vi "fgv_udp_remote.vi"(7 "cmd":enum16{"init", "read", "write", "close"}(ring), 8 "error in":errorcluster, 10 "send data":string) -> (0 "error out":errorcluster, 3 "receive":string)   [LabVIEW 2019]
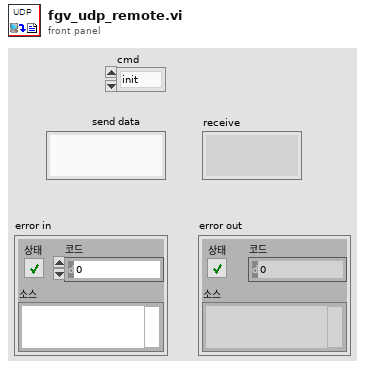
[diagram p1: front panel]
types:
  T1 = cluster{"local port":u16, "remote port":u16, "RBA IP":string}
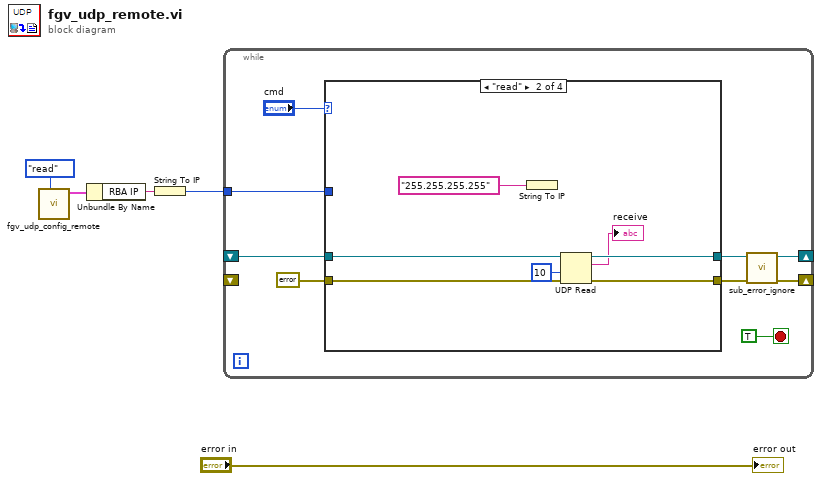
[diagram p0: block diagram]
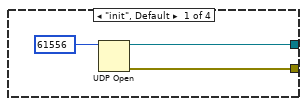
[diagram p2: hidden frame]
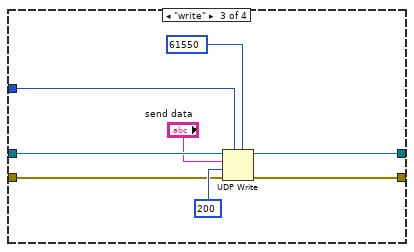
[diagram p3: hidden frame]
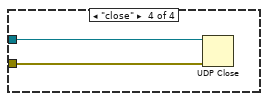
[diagram p4: hidden frame]
diagram:
  n1 = call "fgv_udp_config_remote.vi"("cmd"=enum16{"write", "read"}."read") -> ("udp cfg out"=w3:T1)  [unwired: 9 in, 1 out]
  n2 = Unbundle By Name(w3) -> ("RBA IP"=w4:string)
  n3 = String To IP(1:w4) -> (0:w1:u32)
  n4 = while {
    shift-right: [w11] -> _
    shift-left: _ -> [w10]
    shift-right: [w8] -> _
    shift-left: _ -> [_]
    tunnel: w1 -> [w7]
    stop <- TRUE stop-if-true
    n5 = case shown="\"read\"" "cmd" {
      tunnel: [w16 w22 w28 _] -> w11
      tunnel: [w15 w21 w29 _] -> w9
      tunnel: w10 -> [_ w23 w27 w33]
      tunnel: errorcluster {"status"=FALSE, "code"=0, "source"=""} ("error out") -> [_ w20 w30 w32]
      tunnel: w7 -> [_ _ w24 _]
      frame "init", Default {
        n6 = UDP Open(11:u16 61556 ("포트")) -> (port=w16:refnum<k16>, 0:w15:errorcluster)  [unwired: 4 in, 1 out]
      }
      frame "read" {
        n7 = String To IP(1:"255.255.255.255" ("name")) -> ()  [unwired: 1 out]
        n8 = UDP Read(connection ID=w23, timeout ms (25000)=10 ("타임아웃 ms (25000)"), 8:w20) -> (data out=→"receive":string, error out=w21:errorcluster, 3:w22:refnum<k16>)  [unwired: 1 in, 2 out]
      }
      frame "write" {
        n9 = UDP Write(address=w24, port or service name=u16 61550 ("port"), connection ID=w27, data in="send data", 8:w30, 9:200 ("타임아웃 ms (25000)")) -> (error out=w29:errorcluster, 3:w28:refnum<k16>)
      }
      frame "close" {
        n10 = UDP Close(connection ID=w33, 8:w32) -> ()  [unwired: 2 out]
      }
    }
    n11 = call "sub_error_ignore.vi"("error in"=w9) -> ("error out"=w8:errorcluster)  [unwired: 10 in]
  }
  "error out" <- "error in"
